vi "SLSC Send Commands.vi"(6 "SLSC Dynamic Commands":T1[](array[typedef]), 7 "Timeout?":bool, 8 "error in":errorcluster, 9 "Values":dbl[](array[numeric]), 10 "SLSC Module Name":refnum<k21>, 11 "session in":refnum<k21>) -> (0 "error out":errorcluster, 2 "SLSC Module Name":refnum<k21>, 3 "session out":refnum<k21>)   [LabVIEW 2015, in "SLSC CD Engine.lvlib"]
uses:
  SLSC CD Engine.lvlib
  SLSC Dynamic Channel.ctl
  SLSC Datatype.ctl
  <vilib>/SLSC/Execute Phys Chan Command.vi
  <vilib>/SLSC/Execute Device Command.vi
  <vilib>/SLSC/SLSC.lvlib
  SLSC CD Shared/SLSC CD Shared.lvlib
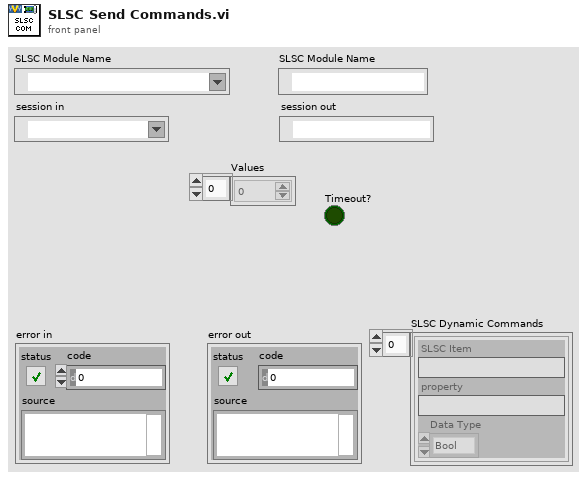
[diagram p1: front panel]
types:
  T1 = typedef "SLSC CD Shared.lvlib/SLSC Dynamic Channel.ctl" = cluster{"SLSC Item":string, "property":string, "Data Type":T2}
  T2 = typedef "SLSC CD Shared.lvlib/SLSC Datatype.ctl" = enum16{"Bool", "Double", "I32", "I64", "String", "U32", "U64"}
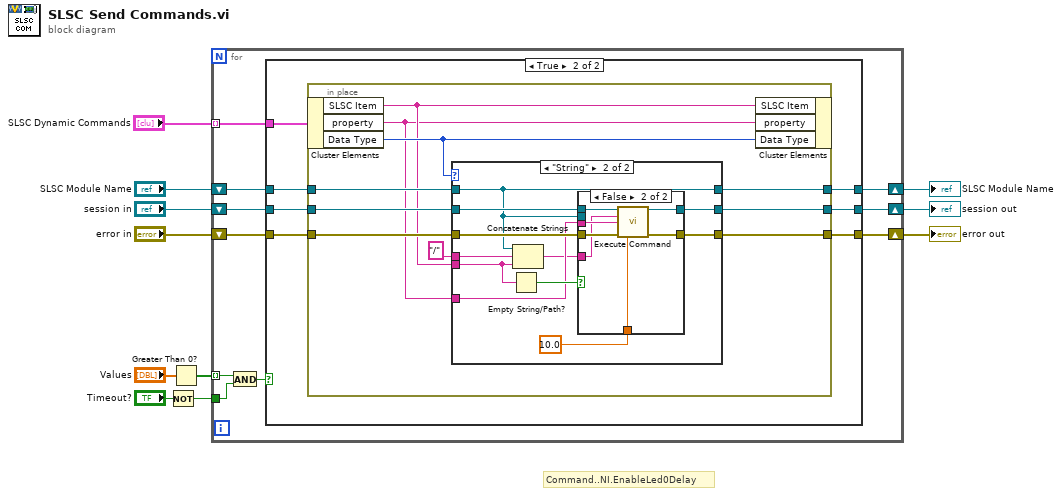
[diagram p0: block diagram]
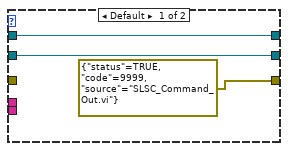
[diagram p3: hidden frame]
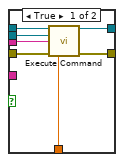
[diagram p4: hidden frame]
diagram:
  # "Command..NI.EnableLed0Delay"
  n1 = Not(x="Timeout?") -> (.not. x?=w1:bool)
  n2 = Greater Than 0?(x="Values") -> (x > 0?=w3:bool[])
  n3 = for {
    tunnel: "SLSC Dynamic Commands" -> [w21] mode=indexing
    shift-right: [w19] -> w6
    shift-left: "session in" -> [w20]
    shift-right: [w17] -> w8
    shift-left: "SLSC Module Name" -> [w18]
    shift-right: [w15] -> w5
    shift-left: "error in" -> [w16]
    tunnel: w3 -> [w14] mode=indexing
    tunnel: w1 -> [w12]
    n4 = And(x=w14, y=w12) -> (x .and. y?=w13:bool)
    n5 = case shown="True" w13 {
      tunnel: w21 -> [_ w25]
      tunnel: w20 -> [w23 w31]
      tunnel: [w23 w30] -> w19
      tunnel: w18 -> [w24 w29]
      tunnel: [w24 w28] -> w17
      tunnel: w16 -> [w22 w27]
      tunnel: [w22 w26] -> w15
      frame False {
      }
      frame True {
        n6 = in-place {
          in-place-border: w31 -> [w41]
          in-place-border: [w40] -> w30
          in-place-border: w29 -> [w39]
          in-place-border: [w38] -> w28
          in-place-border: w27 -> [w37]
          in-place-border: [w36] -> w26
          n7 = in-place-cluster #1(w25) -> ("SLSC Item"=w33:string, "property"=w32:string, "Data Type"=w34:T2)
          n8 = case shown="\"String\"" w34 {
            tunnel: w41 -> [w43 w51]
            tunnel: [w43 w54] -> w40
            tunnel: w33 -> [_ w45]
            tunnel: w39 -> [w44 w48]
            tunnel: [w44 w48] -> w38
            tunnel: w37 -> [_ w50]
            tunnel: [errorcluster {"status"=TRUE, "code"=9999, "source"="SLSC_Command_Out.vi"} ("error out") w53] -> w36
            tunnel: "/" -> [_ w55]
            tunnel: w32 -> [_ w47]
            frame Default {
            }
            frame "String" {
              n9 = Empty String/Path?(string/path=w45) -> (empty?=w49:bool)
              n10 = Concatenate Strings(w48, w55, w45) -> (w46:string)
              n11 = case shown="False" w49 {
                tunnel: w51 -> [w62 w69]
                tunnel: [w61 w68] -> w54
                tunnel: [w60 w67] -> w53
                tunnel: 10.0 ("timeout (10 sec)") -> [w59 w66]
                tunnel: w50 -> [w58 w65]
                tunnel: w47 -> [w57 w64]
                tunnel: w46 -> [_ w63]
                tunnel: w48 -> [w56 _]
                frame True {
                  n12 = call-poly <vilib>:"Execute Command.vi"("session in"=w62, "devices"=w56, "command"=w57, "error in (no error)"=w58, "timeout (10 sec)"=w59) -> ("session out"=w61:refnum<k21>, "error out"=w60:errorcluster)  [unwired: 9 in]
                }
                frame False {
                  n13 = call-poly <vilib>:"Execute Command.vi"("session in"=w69, "physical channels"=w63, "command"=w64, "error in (no error)"=w65, "timeout (10 sec)"=w66) -> ("session out"=w68:refnum<k21>, "error out"=w67:errorcluster)  [unwired: 9 in]
                }
              }
            }
          }
          n14 = in-place-cluster #1("SLSC Item"=w33, "property"=w32, "Data Type"=w34) -> ()  [unwired: 1 out]
        }
      }
    }
  }
  "error out" <- w5
  "session out" <- w6
  "SLSC Module Name" <- w8
